vi "fit.vi"(8 "error in (no error)":errorcluster caption="entrée d'erreur (pas d'erreur)", 11 "Mixture.lvclass 2":refnum<class "Mixture.lvclass">) -> (0 "error out":errorcluster caption="sortie d'erreur", 3 "Mixture.lvclass":refnum<class "Mixture.lvclass">)   [LabVIEW 2020, in "Mixture.lvclass"]
doc: "Estimate model parameters with the EM algorithm.\n\n The method fits the model ``n_init`` times and sets the parameters with\n which the model has the largest likelihood or lower bound. Within each\n trial, the method iterates between E-step and M-step for ``max_iter``\n times until the change of likelihood or lower bound is less than\n ``tol``, otherwise, a ``ConvergenceWarning`` is raised.\n If ``warm_start`` is ``True``, then ``n_init`` is ignored and a single\n initialization is performed upon the first call. Upon consecutive\n calls, training starts where it left off."
uses:
  Mixture.lvclass
  C:/Users/cipop/TDF Dropbox/2_Technologies de France/1 - Services et Etudes/PLAIY/2 - DEV/PLAIYLAB/code/Python/Python.lvclass
  C:/Users/cipop/TDF Dropbox/2_Technologies de France/1 - Services et Etudes/PLAIY/2 - DEV/PLAIYLAB/code/Model/Model.lvclass
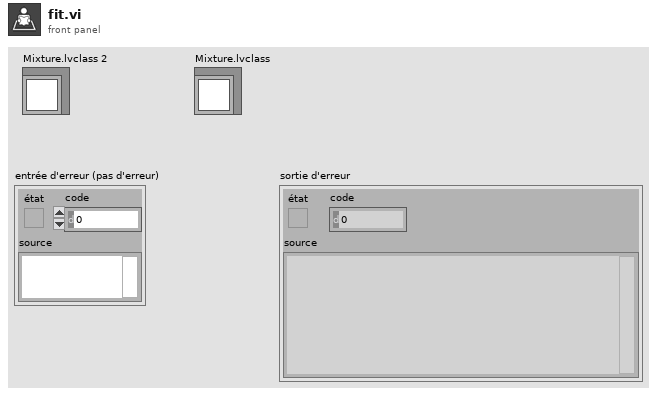
[diagram p1: front panel]
types:
  T1 = typedef "data.ctl" = cluster{"name":string, "X":dbl[][]}
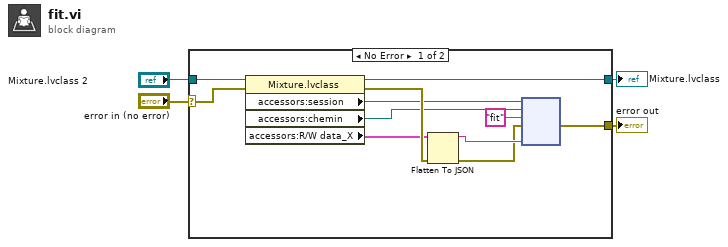
[diagram p0: block diagram]
diagram:
  n1 = case shown="No Error" "error in (no error)" {
    selector: "error in (no error)" -> [w13 w17]
    tunnel: [w14 w17] -> w3
    tunnel: [w6 w16] -> w1
    tunnel: "Mixture.lvclass 2" -> [w5 w16]
    frame No Error {
      n2 = property class="Mixture.lvclass"(reference=w5, error in=w13) -> (reference out=w6:refnum<class "Mixture.lvclass">, error out=w11:errorcluster, "accessors:session"=w8:refnum<k35>, "accessors:chemin"=w7:path, "accessors:R/W data_X"=w9:T1)
      n3 = Flatten To JSON(anything=w9, error in (no error)=w11) -> (JSON string=w12:string, 11:w10:errorcluster)  [unwired: 1 in]
      n4 = node(w8, w7, "fit" ("nom de la fonction"), w10, w12) -> (w14:errorcluster)  [unwired: 3 in, 3 out]
    }
    frame Error {
    }
  }
  "error out" <- w3
  "Mixture.lvclass" <- w1
